vi "Smart IO Get Pwm Input Period Microseconds.vi"(8 "error in (no error)":errorcluster, 11 "deviceIndex":i32) -> (0 "error out":errorcluster, 2 "microseconds out":i32)   [LabVIEW 2026]
doc: "MRC_Status MRC_CALLCONV MRC_SmartIO_GetPwmInputPeriodMicroseconds(int32_t deviceIndex,\n int32_t* microseconds);"
uses:
  MrcLib.lvlib
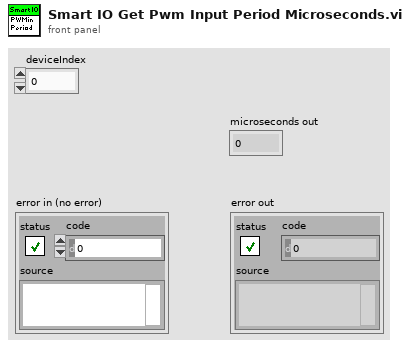
[diagram p1: front panel]
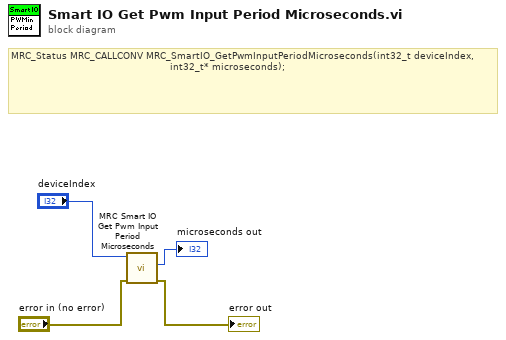
[diagram p0: block diagram]
diagram:
  # "MRC_Status MRC_CALLCONV MRC_SmartIO_GetPwmInputPeriodMicroseconds(int32_t deviceIndex,\n                                                     int32_t* microseconds);"
  n1 = call "MRC Smart IO Get Pwm Input Period Microseconds.vi"("error in (no error)"="error in (no error)", "deviceIndex"="deviceIndex") -> ("error out"=→"error out":errorcluster, "microseconds out"=→"microseconds out":i32)  [unwired: 8 in]
